vi "FT_Close_Device_64bit.vi"(0 "Handle":u64, 11 "error in (no error)":errorcluster) -> (4 "FT_Status":u32(ring) items=["FT_OK", "FT_INVALID_HANDLE", "FT_DEVICE_NOT_FOUND", "FT_DEVICE_NOT_OPENED", "FT_IO_ERROR", "FT_INSUFFICIENT_RESOURCES", "FT_INVALID_PARAMETER", "FT_INVALID_BAUD_RATE", "FT_DEVICE_NOT_OPENED_FOR_ERASE", "FT_DEVICE_NOT_OPENED_FOR_WRITE", "FT_FAILED_TO_WRITE_DEVICE", "FT_EEPROM_READ_FAILED", "FT_EEPROM_WRITE_FAILED", "FT_EEPROM_ERASE_FAILED", "FT_EEPROM_NOT_PRESENT", "FT_EEPROM_NOT_PROGRAMMED", "FT_INVALID_ARGS", "FT_NOT_SUPPORTED", "FT_OTHER_ERROR"], 15 "error out":errorcluster)   [LabVIEW 2019]
uses:
  FTD2XX.dll
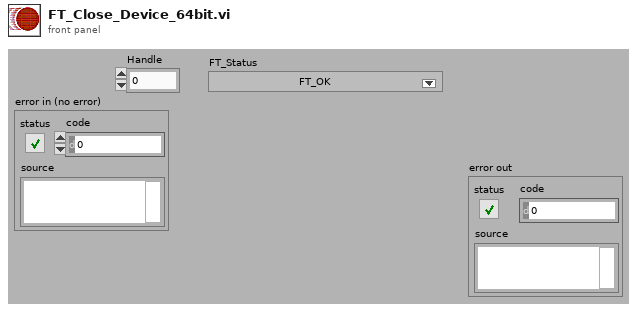
[diagram p1: front panel]
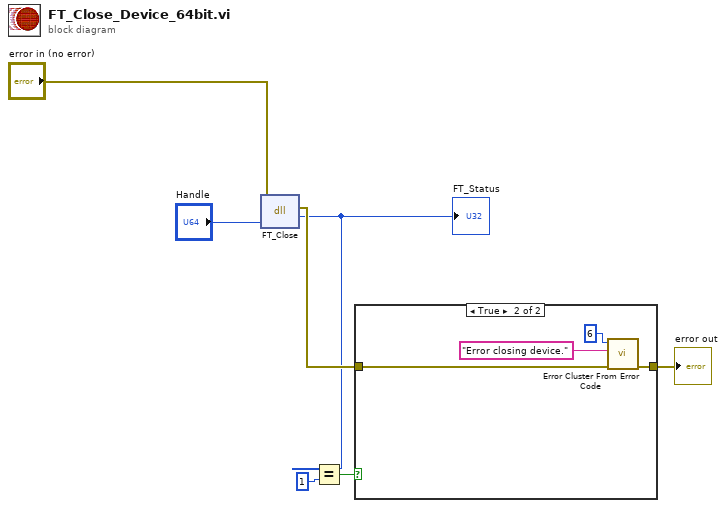
[diagram p0: block diagram]
diagram:
  n1 = dll-call lib="FTD2XX.dll" fn="FT_Close"(error in="error in (no error)", "Handle"="Handle") -> (error out=w2:errorcluster, "FT_Status"=w1:u32)  [unwired: 3 in, 1 out]
  "FT_Status" <- w1
  n2 = Equal?(x=w1, y=u32 1) -> (x = y?=w5:bool)
  n3 = case shown="True" w5 {
    tunnel: [w8 w11] -> w3
    tunnel: w2 -> [w8 w10]
    frame False {
    }
    frame True {
      n4 = call <vilib>:"Error Cluster From Error Code.vi"("error in (no error)"=w10, "error message (\"\")"="Error closing device." ("error message (\"\")"), "error code (0)"=6) -> ("error out"=w11:errorcluster)  [unwired: 6 in]
    }
  }
  "error out" <- w3
